vi "Analog DAQ Configure.vi"(4 "number of samples":i32=1000, 6 "rate":dbl=1000.0 format="%0.2f", 8 "error in":errorcluster, 10 "Canales":tag[](array[tag]), 11 "DAQ Board Name":tag) -> (0 "error out":errorcluster, 3 "task out":refnum<k21>)   [LabVIEW 2020, in "Acquisition .lvlib"]
uses:
  <vilib>/DAQmx/create/channels.llb/DAQmx Create Channel (AI-Voltage-Basic).vi
  <vilib>/DAQmx/configure/timing.llb/DAQmx Timing (Sample Clock).vi
  Acquisition .lvlib
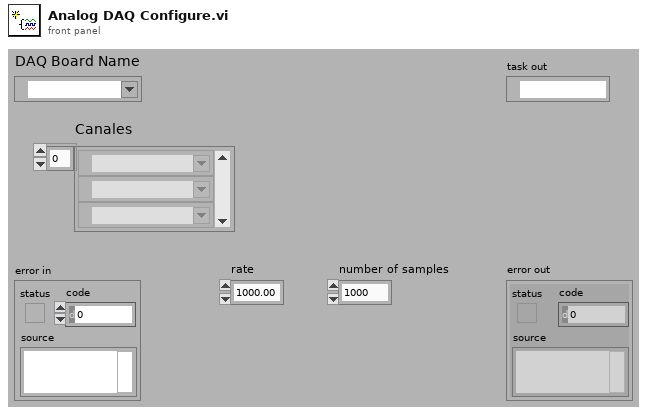
[diagram p1: front panel]
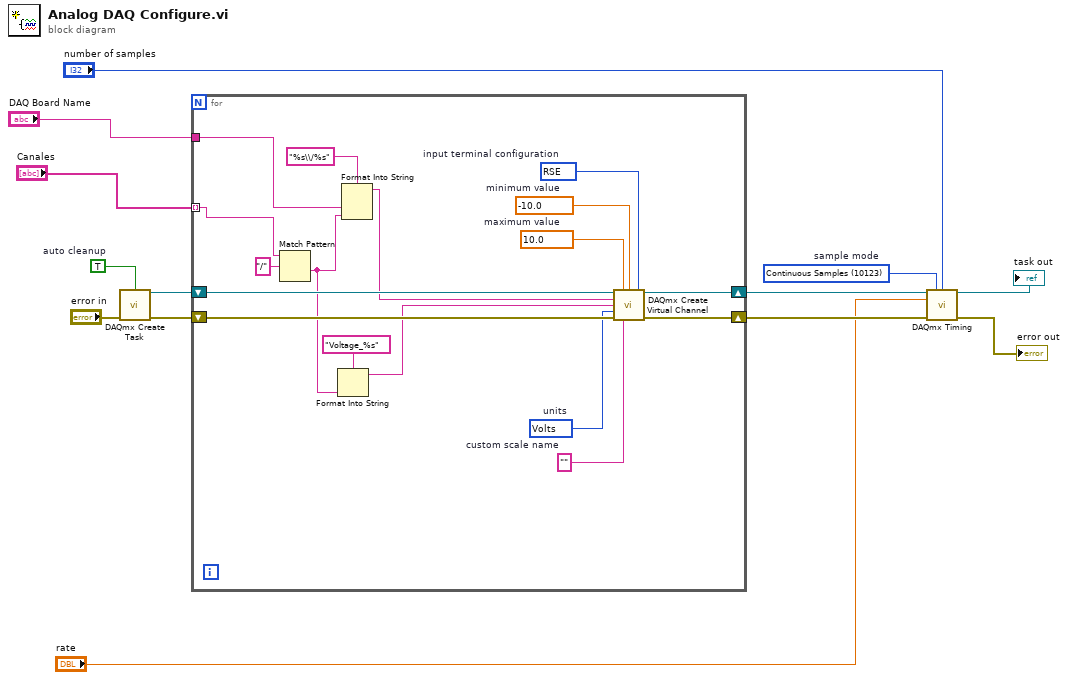
[diagram p0: block diagram]
diagram:
  w4 = 10123 items=["Finite Samples"=10178, "Continuous Samples"=10123, "Hardware Timed Single Point"=12522]  # sample mode
  w11 = TRUE  # auto cleanup
  n1 = call <vilib>:"DAQmx Create Task.vi"("auto cleanup"=w11, "error in"="error in") -> ("task out"=w10:refnum<k21>, "error out"=w12:errorcluster)  [unwired: 12 in]
  n2 = for {
    shift-right: [w25] -> w9
    shift-left: w12 -> [w30]
    shift-right: [w22] -> w8
    shift-left: w10 -> [w29]
    tunnel: "Canales" -> [w14] mode=indexing
    tunnel: "DAQ Board Name" -> [w15]
    w23 = 10083 items=["default"=-1, "RSE"=10083, "NRSE"=10078, "Differential"=10106, "Pseudodifferential"=12529]  # input terminal configuration
    w24 = 10348 items=["Volts"=10348, "From Custom Scale"=10065]  # units
    w26 = ""  # custom scale name
    w27 = -10.0  # minimum value
    w28 = 10.0  # maximum value
    n3 = Match Pattern(string=w14, regular expression="/") -> (after substring=w18:string)  [unwired: 1 in, 3 out]
    n4 = Format Into String(format string="Voltage_%s", w18) -> (resulting string=w19:string)  [unwired: 2 in, 1 out]
    n5 = Format Into String(format string="%s\\/%s", w15, w18) -> (resulting string=w17:string)  [unwired: 2 in, 1 out]
    n6 = call-poly <vilib>:"DAQmx Create Virtual Channel.vi"("task in"=w29, "maximum value"=w28, "minimum value"=w27, "input terminal configuration"=w23, "physical channels"=w17, "name to assign"=w19, "units"=w24, "error in"=w30, "custom scale name"=w26) -> ("task out"=w22:refnum<k21>, "error out"=w25:errorcluster)  [unwired: 5 in]
  }
  n7 = call-poly <vilib>:"DAQmx Timing.vi"("task/channels in"=w8, "sample mode"=w4, "samples per channel"="number of samples", "rate"="rate", "error in"=w9) -> ("task out"=→"task out":refnum<k21>, "error out"=→"error out":errorcluster)  [unwired: 9 in]
